vi "MainVandCur(SubVI).vi"(10 "Main CurrentADC":dbl, 11 "Main Voltage ADC":dbl) -> (2 "Current Out":dbl, 3 "Voltage out":dbl)   [LabVIEW 2013]
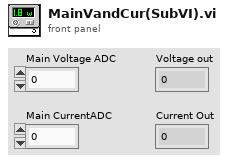
[diagram p1: front panel]
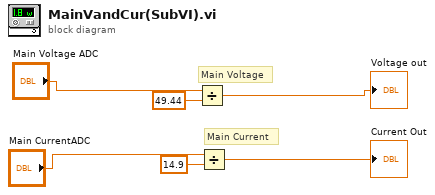
[diagram p0: block diagram]
diagram:
  # "Main Current"
  # "Main Voltage"
  n1 = Divide(x="Main Voltage ADC", y=49.44) -> (x/y=→"Voltage out":dbl)
  n2 = Divide(x="Main CurrentADC", y=14.9) -> (x/y=→"Current Out":dbl)
